vi "qVST.vi"(0 "System no.":i32=1 min=1 max=4 step=1, 5 "error in":errorcluster) -> (14 "Available stages":string[](array[string]), 19 "error out":errorcluster)   [LabVIEW 2020]
doc: "Returns the names of all stages which can be connected to the controller. \n\nC-877, C-884, C-891, E-872, E-873, E-874: Command is available via USB interface only.\n\nC-867, E-871: Command is available via USB, USB DaisyChain or RS232 DaisyChain interface only.\n\nC-887, F-206, M-8X0: Only for GCS syntax version = GCS 2.0 or higher (check with CSV?.vi. If CSV?.vi is not supported, syntax version is GCS 1.0).\n\nMercury_GCS: Command is available via USB interface only."
panel:
  # "Returns the names of all stages which can be connected to the controller."
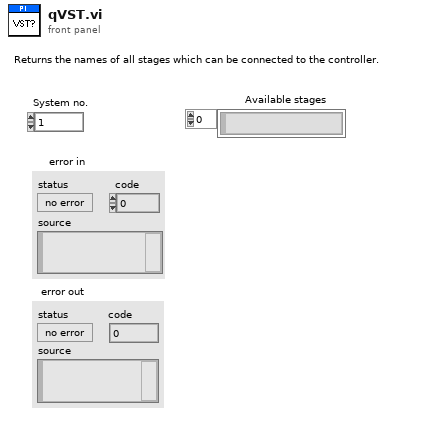
[diagram p1: front panel]
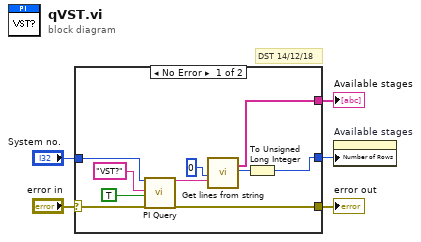
[diagram p0: block diagram]
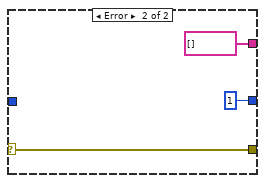
[diagram p2: hidden frame]
diagram:
  # "DST 14/12/18"
  n1 = case shown="No Error" "error in" {
    selector: "error in" -> [w9 w18]
    tunnel: "System no." -> [w13 _]
    tunnel: [w8 string[] [] ("Strings")] -> w4
    tunnel: [w6 u32 1] -> w3
    tunnel: [w10 w18] -> w2
    frame No Error {
      n2 = call "PI Query.vi"("System no."=w13, "String to send"="VST?", "Attach termination char.?"=TRUE ("Attach Linefeed?"), "error in"=w9) -> ("String read"=w11:string, "error out"=w10:errorcluster)  [unwired: 3 in, 11 out]
      n3 = call "Get lines from string.vi"("Array size"=0, "Input string"=w11) -> ("Strings"=w8:string[], "Array size out"=w7:i32)  [unwired: 1 in, 15 out]
      n4 = To Unsigned Long Integer(number=w7) -> (unsigned 32bit integer=w6:u32)
    }
    frame Error {
    }
  }
  "error out" <- w2
  "Available stages" <- w4
  n5 = property on="Available stages" class="Arr (strict)"("Number of Rows"=w3) -> ()  [unwired: 2 in, 2 out]
